vi "Pre Launch Init.vi"(11 "HVAC in":refnum<class "HVAC.lvclass">) -> (0 "error out":errorcluster, 3 "HVAC out":refnum<class "HVAC.lvclass">)   [LabVIEW 2018, in "HVAC Actor.lvlib" / "HVAC.lvclass"]
doc: "(<B>Filename</B>: Actor Framework.lvlib:Actor.lvclass:Pre Launch Init.vi)\n\nDefines behavior that occurs after the Launch Nested Actor method is invoked but before the actor's Actor Core method begins running.\n\nBy default, this method does nothing. A descendant class may override it to define behavior."
uses:
  HVAC.lvclass
  C:/Users/Administrator/Desktop/2018LabVIEW EMS/IED Actors/Device DDS Communications Framework/Device DDS Communications/Device DDS Communications.lvclass
  C:/Users/Administrator/Desktop/2018LabVIEW EMS/EMS Generic Actor/EMS Generic/EMS Generic.lvclass
  Device DDS Communications Framework/Device DDS Communications/Device DDS Communications.lvclass/Device DDS Communications.ctl
  <vilib>/ORNL/CSEISMIC DDS/CSEISMIC DDS Base/CSEISMIC DDS.lvclass/CSEISMIC DDS.ctl
  <vilib>/ORNL/CSEISMIC DDS/CSEISMIC DDS Base/Accessors/Write DDS Reference.vi
  <vilib>/ORNL/CSEISMIC DDS/DDS Writer/DDS Writer.lvclass
  C:/Program Files (x86)/National Instruments/LabVIEW 2018/vi.lib/ORNL/CSEISMIC DDS/CSEISMIC DDS Base/CSEISMIC DDS.lvclass
  <vilib>/ORNL/CSEISMIC DDS/CSEISMIC DDS Base/Error Handler.vi
  Device DDS Communications Framework/Device DDS Communications/Device DDS Communications.lvclass
  EMS Generic Actor/EMS Generic/EMS Generic.lvclass
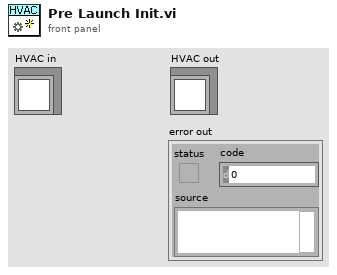
[diagram p1: front panel]
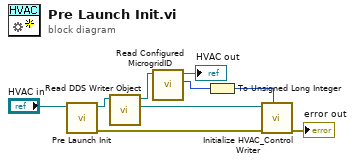
[diagram p0: block diagram]
diagram:
  n1 = call-parent "Pre Launch Init.vi"("Device DDS Communications in"="HVAC in") -> ("error out"=w2:errorcluster, "Device DDS Communications out"=w5:refnum<class "HVAC.lvclass">)  [unwired: 9 in]
  n2 = call "Read DDS Writer Object.vi"("Device DDS Communications in"=w5) -> ("DDS Writer Object"=w9:refnum<class "DDS Writer.lvclass">, "Device DDS Communications out"=w4:refnum<class "HVAC.lvclass">)  [unwired: 9 in]
  n3 = call "Read Configured MicrogridID.vi"("EMS Generic in"=w4) -> ("Microgrid ID"=w8:u8, "EMS Generic out"=→"HVAC out":refnum<class "HVAC.lvclass">)  [unwired: 8 in, 1 out]
  n4 = To Unsigned Long Integer(number=w8) -> (unsigned 32bit integer=w1:u32)
  n5 = call <vilib>:"Initialize HVAC_Control Writer.vi"("MicrogridID"=w1, "error in"=w2, "DDS Writer in"=w9) -> ("error out"=→"error out":errorcluster)  [unwired: 7 in, 1 out]
